vi "Get Multi.vi"(0 "Display State In":T1, 5 "Value In":bool, 9 "Container State":T2, 11 "error in (no error)":errorcluster) -> (4 "Display State Out":T1, 7 "Value Out":bool, 8 "mixed":bool, 15 "error out":errorcluster)   [LabVIEW 2015, in "KCheckbox.xctl"]
uses:
  KCheckbox.xctl
  <vilib>/_xctls/Container State.ctl
  State.ctl
  <vilib>/_xctls/XControlSupport.lvlib
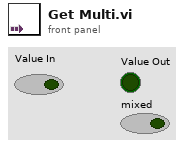
[diagram p1: front panel]
types:
  T1 = typedef "KCheckbox.xctl/State.ctl" = cluster{"mixed":bool, "Value":bool, "update":bool}
  T2 = typedef "XControlSupport.lvlib/Container State.ctl" = cluster{"Indicator?":bool, "Run Mode?":bool, " Refnum":refnum<vi>}
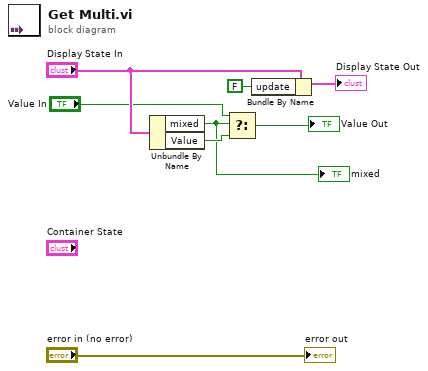
[diagram p0: block diagram]
diagram:
  n1 = Unbundle By Name("Display State In") -> ("mixed"=w1:bool, "Value"=w5:bool)
  "mixed" <- w1
  n2 = Select(t="Value In", s=w1, f=w5) -> (s? t:f=→"Value Out":bool)
  n3 = Bundle By Name(cluster="Display State In", "update"=FALSE) -> (→"Display State Out":T1)
  "error out" <- "error in (no error)"
